vi "move.vi"(2 "Numeric":i32, 3 "Cluster 2":T1) -> (0 "Boolean":bool, 1 "Cluster 3":T1)   [LabVIEW 2014]
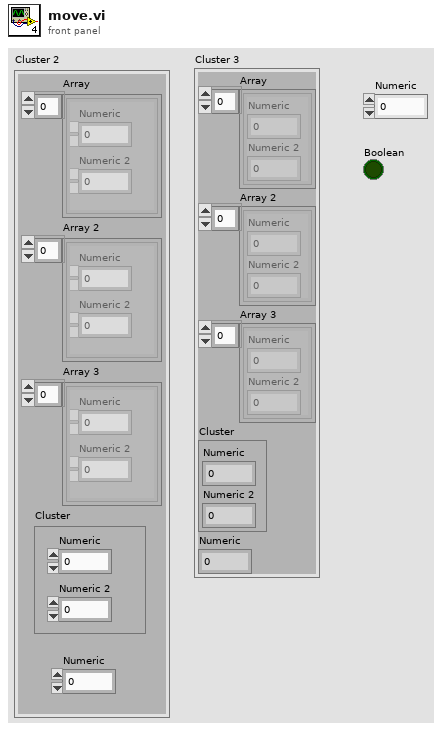
[diagram p1: front panel]
types:
  T1 = cluster{"Array":cluster{"Numeric":dbl, "Numeric 2":dbl}[], "Array 2":cluster{"Numeric":dbl, "Numeric 2":dbl}[], "Array 3":cluster{"Numeric":dbl, "Numeric 2":dbl}[], "Cluster":cluster{"Numeric":dbl, "Numeric 2":dbl}, "Numeric":dbl}
  T2 = cluster{"Array":cluster{"Numeric":dbl, "Numeric 2":dbl}[], "Array 2":cluster{"Numeric":dbl, "Numeric 2":dbl}[], "Array 3":cluster{"Numeric":dbl, "Numeric 2":dbl}[], cluster{"Numeric":dbl, "Numeric 2":dbl}, dbl}
  T3 = cluster{"Array":cluster{"Numeric":dbl, "Numeric 2":dbl}[], "Array 2":cluster{"Numeric":dbl, "Numeric 2":dbl}[], cluster{"Numeric":dbl, "Numeric 2":dbl}[], cluster{"Numeric":dbl, "Numeric 2":dbl}, dbl}
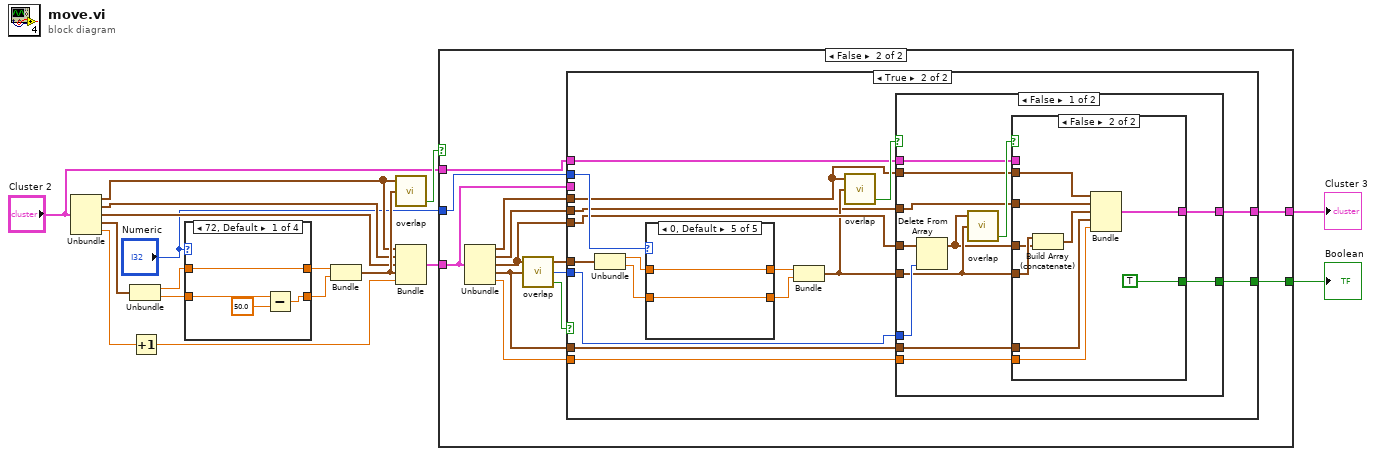
[diagram p0: block diagram]
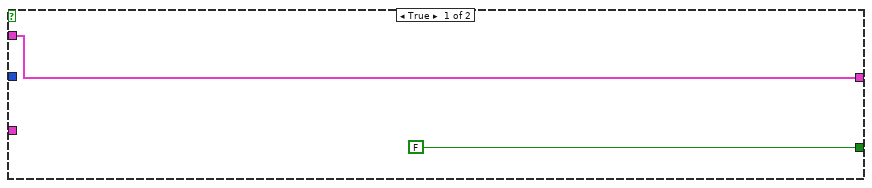
[diagram p2: hidden frame]
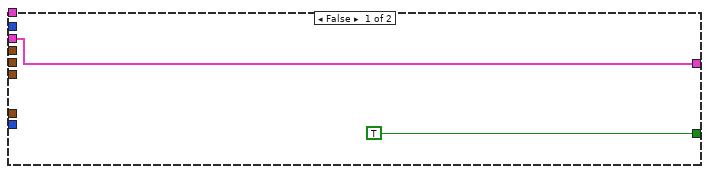
[diagram p3: hidden frame]
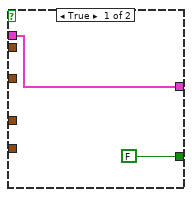
[diagram p4: hidden frame]
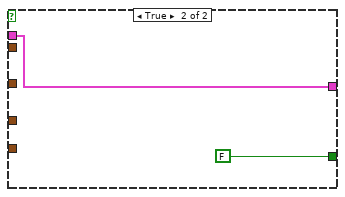
[diagram p5: hidden frame]
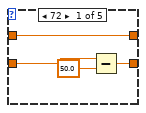
[diagram p6: hidden frame]
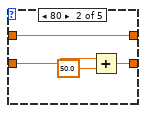
[diagram p7: hidden frame]
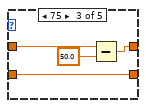
[diagram p8: hidden frame]
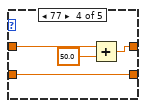
[diagram p9: hidden frame]
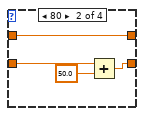
[diagram p10: hidden frame]
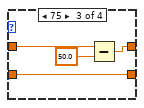
[diagram p11: hidden frame]
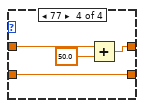
[diagram p12: hidden frame]
diagram:
  n1 = Unbundle("Cluster 2") -> ("Array"=w9:cluster{"Numeric":dbl, "Numeric 2":dbl}[], "Array 2"=w8:cluster{"Numeric":dbl, "Numeric 2":dbl}[], "Array 3"=w7:cluster{"Numeric":dbl, "Numeric 2":dbl}[], "Cluster"=w14:cluster{"Numeric":dbl, "Numeric 2":dbl}, "Numeric"=w10:dbl)
  n2 = Unbundle(w14) -> ("Numeric"=w17:dbl, "Numeric 2"=w16:dbl)
  n3 = Increment(x=w10) -> (x+1=w11:dbl)
  n4 = case shown="72, Default" "Numeric" {
    tunnel: w17 -> [w20 w24 w28 w32]
    tunnel: w16 -> [w21 w25 w27 w31]
    tunnel: [w20 w24 w29 w33] -> w13
    tunnel: [w19 w23 w27 w31] -> w15
    frame 72, Default {
      n5 = Subtract(x=w21, y=50.0) -> (x-y=w19:dbl)
    }
    frame 80 {
      n6 = Add(x=w25, y=50.0) -> (x+y=w23:dbl)
    }
    frame 75 {
      n7 = Subtract(x=w28, y=50.0) -> (x-y=w29:dbl)
    }
    frame 77 {
      n8 = Add(x=w32, y=50.0) -> (x+y=w33:dbl)
    }
  }
  n9 = Bundle("Numeric"=w13, "Numeric 2"=w15) -> (w12:cluster{"Numeric":dbl, "Numeric 2":dbl})  [unwired: 1 in]
  n10 = call "overlap.vi"("Cluster"=w12, "Array"=w9) -> ("Boolean"=w6:bool)  [unwired: 1 in, 2 out]
  n11 = Bundle("Array"=w9, "Array 2"=w8, "Array 3"=w7, w12, w11) -> (w5:T2)  [unwired: 1 in]
  n12 = case shown="False" w6 {
    tunnel: "Cluster 2" -> [w35 w39]
    tunnel: w5 -> [_ w43]
    tunnel: "Numeric" -> [_ w38]
    tunnel: [w35 w37] -> w2
    tunnel: [FALSE w36] -> w3
    frame True {
    }
    frame False {
      n13 = Unbundle(w43) -> ("Array"=w44:cluster{"Numeric":dbl, "Numeric 2":dbl}[], "Array 2"=w45:cluster{"Numeric":dbl, "Numeric 2":dbl}[], "Array 3"=w42:cluster{"Numeric":dbl, "Numeric 2":dbl}[], w41:cluster{"Numeric":dbl, "Numeric 2":dbl}, w40:dbl)
      n14 = call "overlap.vi"("Cluster"=w41, "Array"=w42) -> ("Boolean"=w48:bool, "Numeric"=w46:i32, "Cluster 2"=w47:cluster{"Numeric":dbl, "Numeric 2":dbl})  [unwired: 1 in]
      n15 = case shown="True" w48 {
        tunnel: w47 -> [_ w63]
        tunnel: w46 -> [_ w59]
        tunnel: w45 -> [_ w57]
        tunnel: w44 -> [_ w56]
        tunnel: w43 -> [w49 _]
        tunnel: w42 -> [_ w60]
        tunnel: w41 -> [_ w55]
        tunnel: w40 -> [_ w54]
        tunnel: w39 -> [_ w53]
        tunnel: w38 -> [_ w62]
        tunnel: [w49 w52] -> w37
        tunnel: [TRUE w51] -> w36
        frame False {
        }
        frame True {
          n16 = Unbundle(w63) -> ("Numeric"=w64:dbl, "Numeric 2"=w65:dbl)
          n17 = case shown="0, Default" w62 {
            tunnel: w64 -> [w95 w99 w103 w107 w110]
            tunnel: w65 -> [w96 w100 w102 w106 w109]
            tunnel: [w95 w99 w104 w108 w110] -> w67
            tunnel: [w94 w98 w102 w106 w109] -> w66
            frame 72 {
              n18 = Subtract(x=w96, y=50.0) -> (x-y=w94:dbl)
            }
            frame 80 {
              n19 = Add(x=w100, y=50.0) -> (x+y=w98:dbl)
            }
            frame 75 {
              n20 = Subtract(x=w103, y=50.0) -> (x-y=w104:dbl)
            }
            frame 77 {
              n21 = Add(x=w107, y=50.0) -> (x+y=w108:dbl)
            }
            frame 0, Default {
            }
          }
          n22 = Bundle("Numeric"=w67, "Numeric 2"=w66) -> (w58:cluster{"Numeric":dbl, "Numeric 2":dbl})  [unwired: 1 in]
          n23 = call "overlap.vi"("Cluster"=w58, "Array"=w56) -> ("Boolean"=w61:bool)  [unwired: 1 in, 2 out]
          n24 = case shown="False" w61 {
            tunnel: w60 -> [w79 _]
            tunnel: w59 -> [w78 _]
            tunnel: w58 -> [w76 _]
            tunnel: w57 -> [w73 _]
            tunnel: w56 -> [w74 _]
            tunnel: w55 -> [w72 _]
            tunnel: w54 -> [w71 _]
            tunnel: w53 -> [w70 w91]
            tunnel: [w69 w91] -> w52
            tunnel: [w68 FALSE] -> w51
            frame False {
              n25 = Delete From Array(array=w79, index=w78) -> (array with subset deleted=w75:cluster{"Numeric":dbl, "Numeric 2":dbl}[])  [unwired: 1 in, 1 out]
              n26 = call "overlap.vi"("Cluster"=w76, "Array"=w75) -> ("Boolean"=w77:bool)  [unwired: 1 in, 2 out]
              n27 = case shown="False" w77 {
                tunnel: w76 -> [_ w90]
                tunnel: w75 -> [_ w89]
                tunnel: w74 -> [_ w86]
                tunnel: w73 -> [_ w87]
                tunnel: w72 -> [_ w85]
                tunnel: w71 -> [_ w84]
                tunnel: w70 -> [w80 _]
                tunnel: [w80 w83] -> w69
                tunnel: [FALSE TRUE] -> w68
                frame True {
                }
                frame False {
                  n28 = Build Array (concatenate)(w90, w89) -> (w88:cluster{"Numeric":dbl, "Numeric 2":dbl}[])
                  n29 = Bundle("Array"=w86, "Array 2"=w87, w88, w85, w84) -> (w83:T3)  [unwired: 1 in]
                }
              }
            }
            frame True {
            }
          }
        }
      }
    }
  }
  "Cluster 3" <- w2
  "Boolean" <- w3
